vi "Wait.vi"   [LabVIEW 2016, in "Aerotech VIs.lvlib"]
uses:
  Aerotech VIs.lvlib
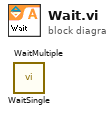
[diagram p0: block diagram]
diagram:
  n1 = call "WaitMultiple.vi"() -> ()  [unwired: 9 in, 3 out]
  n2 = call "WaitSingle.vi"() -> ()  [unwired: 9 in, 3 out]
